vi "SignalObservation_HT.vi"(6 "error in (no error)":errorcluster, 9 "Signal":string(combo)="ObsClk") -> (0 "error out":errorcluster)   [LabVIEW 2011]
doc: "This VI outputs a selected signal from the HT Link 0 PLL.\n\nInputs:\n1. Signal: PLL Clock to output (Refclk, VCO, etc.)."
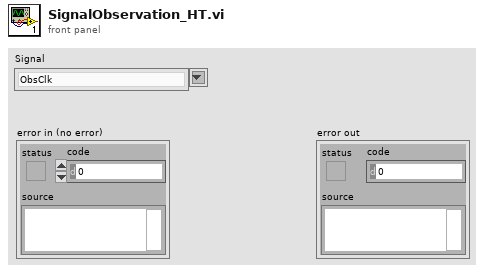
[diagram p1: front panel]
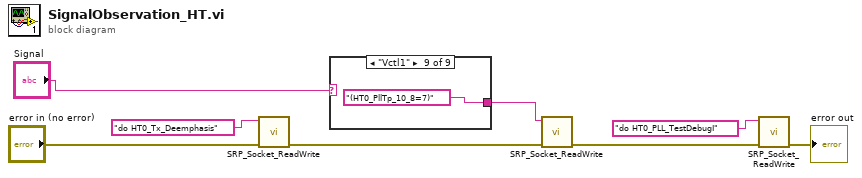
[diagram p0: block diagram]
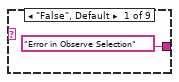
[diagram p2: hidden frame]
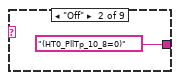
[diagram p3: hidden frame]
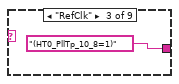
[diagram p4: hidden frame]
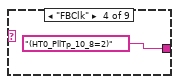
[diagram p5: hidden frame]
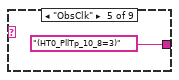
[diagram p6: hidden frame]
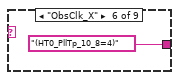
[diagram p7: hidden frame]
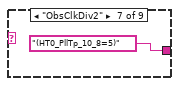
[diagram p8: hidden frame]
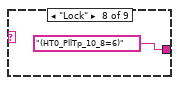
[diagram p9: hidden frame]
diagram:
  n1 = call "SRP_Socket_ReadWrite.vi"("error in (no error)"="error in (no error)", "Data In"="do HT0_Tx_Deemphasis") -> ("error out"=w6:errorcluster)  [unwired: 7 in, 1 out]
  n2 = case shown="\"Vctl1\"" "Signal" {
    tunnel: ["Error in Observe Selection" "(HT0_PllTp_10_8=0)" "(HT0_PllTp_10_8=1)" "(HT0_PllTp_10_8=2)" "(HT0_PllTp_10_8=3)" "(HT0_PllTp_10_8=4)" "(HT0_PllTp_10_8=5)" "(HT0_PllTp_10_8=6)" "(HT0_PllTp_10_8=7)"] -> w3
    frame "False", Default {
    }
    frame "Off" {
    }
    frame "RefClk" {
    }
    frame "FBClk" {
    }
    frame "ObsClk" {
    }
    frame "ObsClk_X" {
    }
    frame "ObsClkDiv2" {
    }
    frame "Lock" {
    }
    frame "Vctl1" {
    }
  }
  n3 = call "SRP_Socket_ReadWrite.vi"("error in (no error)"=w6, "Data In"=w3) -> ("error out"=w5:errorcluster)  [unwired: 7 in, 1 out]
  n4 = call "SRP_Socket_ReadWrite.vi"("error in (no error)"=w5, "Data In"="do HT0_PLL_TestDebugI") -> ("error out"=→"error out":errorcluster)  [unwired: 7 in, 1 out]
